vi "SEQ Write DVR.vi"(7 "Module Name":string, 8 "error in (no error)":errorcluster, 11 "data value reference":refnum<data-value>) -> (0 "error out":errorcluster)   [LabVIEW 2019, in "ADLINK Motion Card.lvlib"]
uses:
  ADLINK Motion Card.lvlib
  SEQ/SEQ Data.ctl
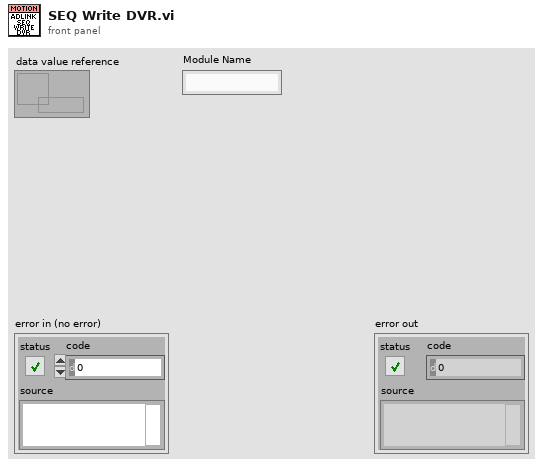
[diagram p1: front panel]
types:
  T1 = typedef "ADLINK Motion Card.lvlib/SEQ Data.ctl" = cluster{"Current Position":dbl, "Target Position":dbl, "Velocity":dbl, "Acceleration":dbl, "Arrived?":bool, "data value reference":refnum<data-value>, "VI Refnum":refnum<vi>}
  T2 = cluster{"Current Position":dbl, "Target Position":dbl, "Velocity":dbl, "Acceleration":dbl, "Arrived?":bool}
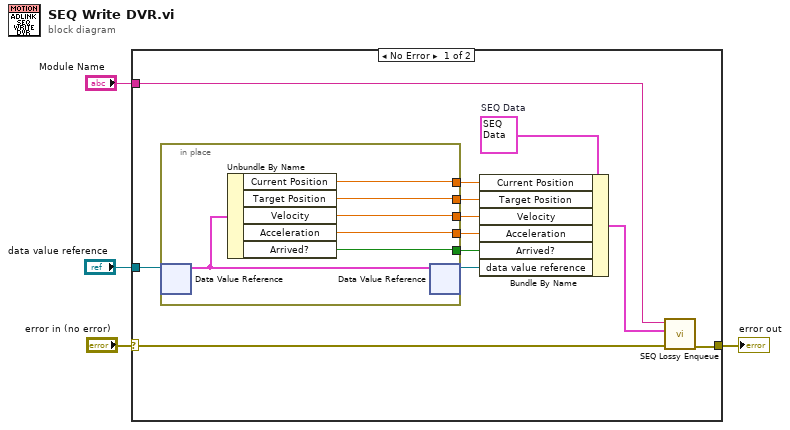
[diagram p0: block diagram]
diagram:
  n1 = case shown="No Error" "error in (no error)" {
    selector: "error in (no error)" -> [w7 w23]
    tunnel: "Module Name" -> [w8 _]
    tunnel: "data value reference" -> [w16 _]
    tunnel: [w6 w23] -> w1
    frame No Error {
      w14 = T1 {"Current Position"=0.0, "Target Position"=0.0, "Velocity"=0.0, "Acceleration"=0.0, "Arrived?"=FALSE, "data value reference"=refnum, "VI Refnum"=refnum}  # SEQ Data
      n2 = in-place {
        in-place-border: [w22] -> w13
        in-place-border: [w21] -> w12
        in-place-border: [w20] -> w11
        in-place-border: [w19] -> w10
        in-place-border: [w18] -> w9
        n3 = in-place-dvr #1(w16) -> (w17:T2)  [unwired: 1 out]
        n4 = Unbundle By Name(w17) -> ("Current Position"=w22:dbl, "Target Position"=w21:dbl, "Velocity"=w20:dbl, "Acceleration"=w19:dbl, "Arrived?"=w18:bool)
        n5 = in-place-dvr #1(w17) -> (w5:refnum<data-value>)  [unwired: 1 out]
      }
      n6 = Bundle By Name(cluster=w14, "Current Position"=w13, "Target Position"=w12, "Velocity"=w11, "Acceleration"=w10, "Arrived?"=w9, "data value reference"=w5) -> (w15:T1)
      n7 = call "SEQ Lossy Enqueue.vi"("error in (no error)"=w7, "Setting"=w15, "Queue Name"=w8) -> ("error out"=w6:errorcluster)  [unwired: 8 in]
    }
    frame Error {
    }
  }
  "error out" <- w1
